vi "Get Manipulator Displacements.vi"(6 "Transformation Matrix":T1, 7 "Scale Coorection Factor":cluster{"Kx":dbl, "Ky":dbl, "Kz":dbl}={"Kx"=-0.030159441585130214, "Ky"=0.5585990541241189, "Kz"=-0.030159441585130214}, 9 "Angles":cluster{"phi [rad]":dbl, "theta [rad]":dbl}, 10 "Target Coordinates":T2, 11 "Tip Coordinates":T2) -> (1 "Error":bool, 2 "Approach Step":dbl format="%.2f", 3 "Manipulator Displacements":T2 {"X" format="%.2f"; "Y" format="%.2f"; "Z" format="%.2f"})   [LabVIEW 2012, in "Targeting Unit.lvlib"]
uses:
  Targeting Unit.lvlib
  <vilib>/Analysis/Matrix/Datatypes/RealMatrix.ctl
  <vilib>/Analysis/Matrix/NI_Matrix.lvlib
panel:
  # "X entering (1) or exiting tip (-1)"
  # "Flip (Yes -1 No 1)"
  # "Insertion step coefficient"
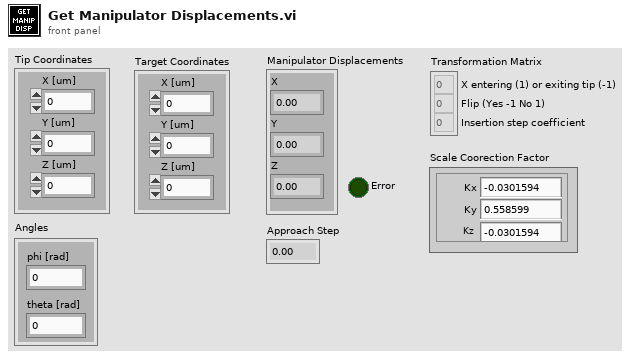
[diagram p1: front panel]
types:
  T1 = typedef "NI_Matrix.lvlib/RealMatrix.ctl" = dbl[][]
  T2 = cluster{"X [um]":dbl, "Y [um]":dbl, "Z [um]":dbl}
  T3 = cluster{"X [um]":bool, "Y [um]":bool, "Z [um]":bool}
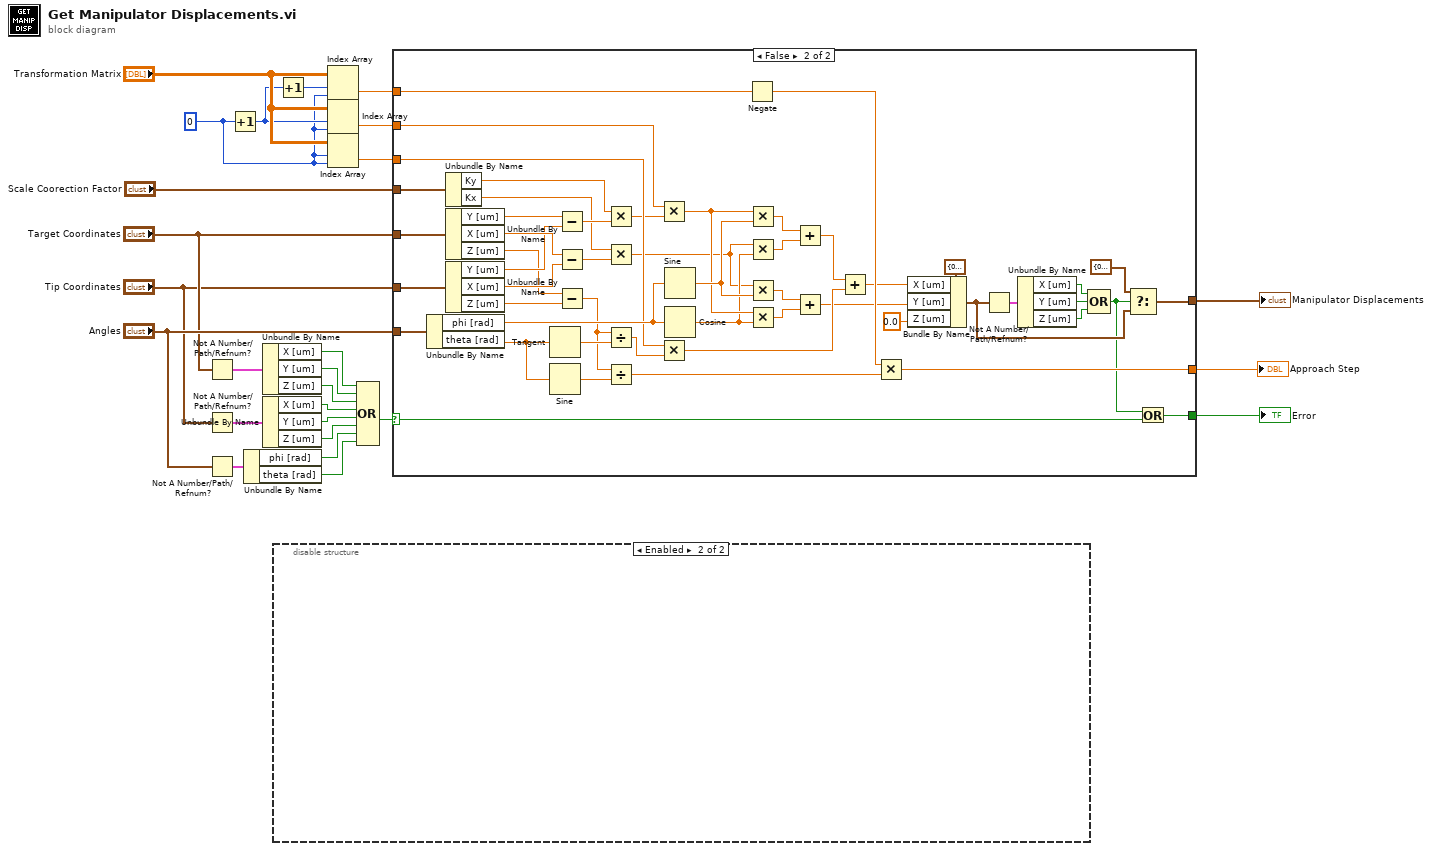
[diagram p0: block diagram]
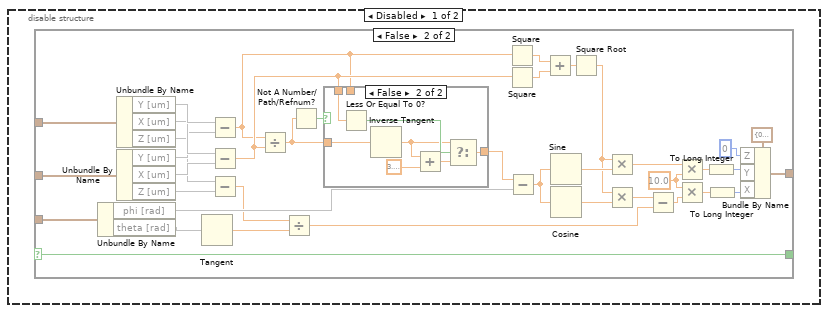
[diagram p2: hidden frame]
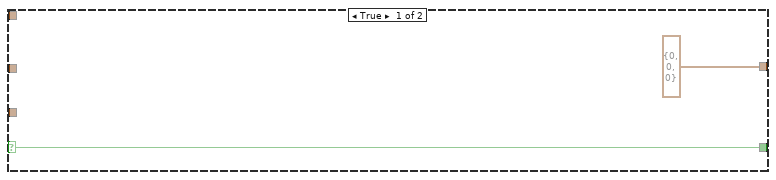
[diagram p3: hidden frame]
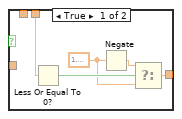
[diagram p4: hidden frame]
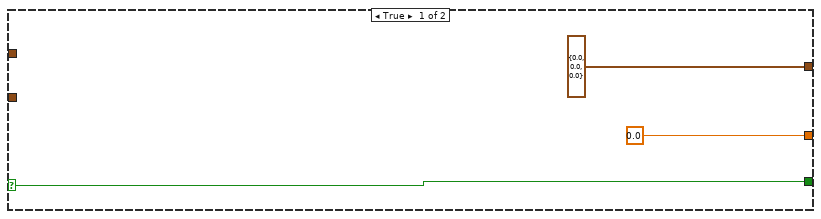
[diagram p5: hidden frame]
diagram:
  w2 = 0 ("index (col)")
  n1 = Not A Number/Path/Refnum?(number/path/refnum="Target Coordinates") -> (NaN/Path/Refnum?=w26:T3)
  n2 = Not A Number/Path/Refnum?(number/path/refnum="Tip Coordinates") -> (NaN/Path/Refnum?=w25:T3)
  n3 = Not A Number/Path/Refnum?(number/path/refnum="Angles") -> (NaN/Path/Refnum?=w24:cluster{"phi [rad]":bool, "theta [rad]":bool})
  n4 = Increment(x=w2) -> (x+1=w10:i32)
  n5 = Unbundle By Name(w24) -> ("phi [rad]"=w20:bool, "theta [rad]"=w21:bool)
  n6 = Unbundle By Name(w26) -> ("X [um]"=w15:bool, "Y [um]"=w16:bool, "Z [um]"=w17:bool)
  n7 = Unbundle By Name(w25) -> ("X [um]"=w18:bool, "Y [um]"=w19:bool, "Z [um]"=w14:bool)
  n8 = disable-structure shown="Enabled" {
    frame Disabled {
      n9 = case shown="False" {
        selector: _ -> [w27 w33]
        tunnel: _ -> [_ w37]
        tunnel: _ -> [_ w36]
        tunnel: _ -> [_ w35]
        tunnel: [cluster{"X":i32, "Y":i32, "Z":i32} {"X"=0, "Y"=0, "Z"=0} ("input cluster") w34] -> _
        tunnel: [w27 w33] -> _
        frame True {
        }
        frame False {
          w39 = 10.0 ("Z")
          n10 = Unbundle By Name(w36) -> ("phi [rad]"=w63, "theta [rad]"=w58)
          n11 = Unbundle By Name(w35) -> ("Y [um]"=w66, "X [um]"=w65, "Z [um]"=w44)
          n12 = Unbundle By Name(w37) -> ("Y [um]"=w47, "X [um]"=w51, "Z [um]"=w43)
          n13 = Tangent(1:w58) -> (0:w45:dbl)
          n14 = Subtract(x=w66, y=w47) -> (x-y=w29:dbl)
          n15 = Subtract(x=w65, y=w51) -> (x-y=w32:dbl)
          n16 = Subtract(x=w44, y=w43) -> (x-y=w46:dbl)
          n17 = Divide(x=w29, y=w32) -> (x/y=w31:dbl)
          n18 = Divide(x=w46, y=w45) -> (x/y=w64:dbl)
          n19 = Not A Number/Path/Refnum?(number/path/refnum=w31) -> (NaN/Path/Refnum?=w30:bool)
          n20 = case shown="False" w30 {
            tunnel: [w70 w78] -> w54
            tunnel: w32 -> [_ w73]
            tunnel: w31 -> [_ w72]
            tunnel: w29 -> [w71 _]
            frame True {
              w67 = 1.5707963267948966
              n21 = Less Or Equal To 0?(x=w71) -> (x <= 0?=w69:bool)
              n22 = Negate(x=w67) -> (-x=w68:dbl)
              n23 = Select(t=w68, s=w69, f=w67) -> (s? t:f=w70:dbl)
            }
            frame False {
              n24 = Less Or Equal To 0?(x=w73) -> (x <= 0?=w77:bool)
              n25 = Inverse Tangent(1:w72) -> (0:w76:dbl)
              n26 = Add(x=w76, y=3.141592653589793) -> (x+y=w74:dbl)
              n27 = Select(t=w76, s=w77, f=w74) -> (s? t:f=w78:dbl)
            }
          }
          n28 = Square(x=w29) -> (x^2=w48:dbl)
          n29 = Square(x=w32) -> (x^2=w49:dbl)
          n30 = Subtract(x=w54, y=w63) -> (x-y=w53:dbl)
          n31 = Add(x=w48, y=w49) -> (x+y=w50:dbl)
          n32 = Sine(x=w53) -> (sin(x)=w57:dbl)
          n33 = Cosine(x=w53) -> (cos(x)=w59:dbl)
          n34 = Square Root(x=w50) -> (sqrt(x)=w52:dbl)
          n35 = Multiply(x=w52, y=w57) -> (x*y=w42:dbl)
          n36 = Multiply(x=w52, y=w59) -> (x*y=w60:dbl)
          n37 = Subtract(x=w60, y=w64) -> (x-y=w61:dbl)
          n38 = Multiply(x=w42, y=w39) -> (x*y=w40:dbl)
          n39 = Multiply(x=w39, y=w61) -> (x*y=w41:dbl)
          n40 = To Long Integer(number=w40) -> (32bit integer=w56:i32)
          n41 = To Long Integer(number=w41) -> (32bit integer=w62:i32)
          n42 = Bundle By Name(cluster=cluster{"X":i32, "Y":i32, "Z":i32} {"X"=0, "Y"=0, "Z"=0} ("input cluster"), "Z"=0, "Y"=w56, "X"=w62) -> (w34:cluster{"X":i32, "Y":i32, "Z":i32})
        }
      }
    }
    frame Enabled {
    }
  }
  n43 = Increment(x=w10) -> (x+1=w3:i32)
  n44 = Index Array(array="Transformation Matrix", index (row)=w3, index (col)=w2) -> (element=w7:dbl)
  n45 = Index Array(array="Transformation Matrix", index (row)=w10, index (col)=w2) -> (element=w9:dbl)
  n46 = Index Array(array="Transformation Matrix", index (row)=w2, index (col)=w2) -> (element=w8:dbl)
  n47 = Compound Arithmetic op=OR(w15, w16, w17, w18, w19, w14, w20, w21) -> (w23:bool)
  n48 = case shown="False" w23 {
    selector: w23 -> [w80 w90]
    tunnel: "Tip Coordinates" -> [_ w125]
    tunnel: "Angles" -> [_ w124]
    tunnel: "Target Coordinates" -> [_ w123]
    tunnel: [cluster{"X":dbl, "Y":dbl, "Z":dbl} {"X"=0.0, "Y"=0.0, "Z"=0.0} ("input cluster") w93] -> w13
    tunnel: [w80 w91] -> w12
    tunnel: w9 -> [_ w112]
    tunnel: w8 -> [_ w111]
    tunnel: w7 -> [_ w104]
    tunnel: [0.0 w101] -> w4
    tunnel: "Scale Coorection Factor" -> [_ w82]
    frame True {
    }
    frame False {
      n49 = Unbundle By Name(w124) -> ("phi [rad]"=w122:dbl, "theta [rad]"=w108:dbl)
      n50 = Unbundle By Name(w82) -> ("Ky"=w84:dbl, "Kx"=w83:dbl)
      n51 = Unbundle By Name(w123) -> ("Y [um]"=w132:dbl, "X [um]"=w131:dbl, "Z [um]"=w127:dbl)
      n52 = Unbundle By Name(w125) -> ("Y [um]"=w129:dbl, "X [um]"=w130:dbl, "Z [um]"=w126:dbl)
      n53 = Tangent(1:w108) -> (0:w128:dbl)
      n54 = Sine(x=w108) -> (sin(x)=w106:dbl)
      n55 = Subtract(x=w132, y=w129) -> (x-y=w87:dbl)
      n56 = Subtract(x=w131, y=w130) -> (x-y=w86:dbl)
      n57 = Subtract(x=w127, y=w126) -> (x-y=w107:dbl)
      n58 = Multiply(x=w84, y=w87) -> (x*y=w88:dbl)
      n59 = Multiply(x=w83, y=w86) -> (x*y=w85:dbl)
      n60 = Divide(x=w107, y=w128) -> (x/y=w114:dbl)
      n61 = Divide(x=w107, y=w106) -> (x/y=w105:dbl)
      n62 = Multiply(x=w112, y=w88) -> (x*y=w116:dbl)
      n63 = Multiply ("Multiply.vi")(x=w111, y=w114) -> (x*y=w113:dbl)
      n64 = Sine(x=w122) -> (sin(x)=w117:dbl)
      n65 = Cosine(x=w122) -> (cos(x)=w115:dbl)
      n66 = Negate(x=w104) -> (-x=w103:dbl)
      n67 = Multiply(x=w116, y=w117) -> (x*y=w121:dbl)
      n68 = Multiply(x=w85, y=w115) -> (x*y=w120:dbl)
      n69 = Multiply(x=w85, y=w117) -> (x*y=w119:dbl)
      n70 = Multiply(x=w116, y=w115) -> (x*y=w118:dbl)
      n71 = Add(x=w121, y=w120) -> (x+y=w109:dbl)
      n72 = Add(x=w119, y=w118) -> (x+y=w99:dbl)
      n73 = Add ("Add.vi")(x=w109, y=w113) -> (x+y=w100:dbl)
      n74 = Multiply ("Multiply.vi")(x=w103, y=w105) -> (x*y=w101:dbl)
      n75 = Bundle By Name(cluster=T2 {"X [um]"=0.0, "Y [um]"=0.0, "Z [um]"=0.0} ("Target Coordinates"), "X [um]"=w100, "Y [um]"=w99, "Z [um]"=0.0 ("Z")) -> (w94:T2)
      n76 = Not A Number/Path/Refnum?(number/path/refnum=w94) -> (NaN/Path/Refnum?=w98:T3)
      n77 = Unbundle By Name(w98) -> ("X [um]"=w97:bool, "Y [um]"=w96:bool, "Z [um]"=w95:bool)
      n78 = Compound Arithmetic op=OR(w97, w96, w95) -> (w89:bool)
      n79 = Select(t=T2 {"X [um]"=0.0, "Y [um]"=0.0, "Z [um]"=0.0}, s=w89, f=w94) -> (s? t:f=w93:T2)
      n80 = Or(x=w89, y=w90) -> (x .or. y?=w91:bool)
    }
  }
  "Manipulator Displacements" <- w13
  "Error" <- w12
  "Approach Step" <- w4
